vi "Resolve Direction Position.vi"(7 "Board Size":i32, 10 "Direction":T1, 11 "From":T2) -> (2 "Col":i32, 3 "Row":i32, 5 "To":T2)   [LabVIEW 2020, in "SquareBattle.lvlib"]
uses:
  SquareBattle.lvlib
  Position.ctl
  Direction.ctl
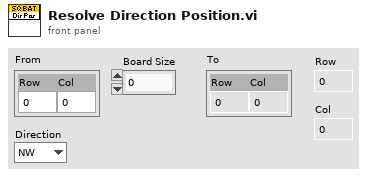
[diagram p1: front panel]
types:
  T1 = typedef "SquareBattle.lvlib/Direction.ctl" = enum16{"NW", "N", "NE", "E", "SE", "S", "SW", "W"}
  T2 = typedef "SquareBattle.lvlib/Position.ctl" = cluster{"Row":i32, "Col":i32}
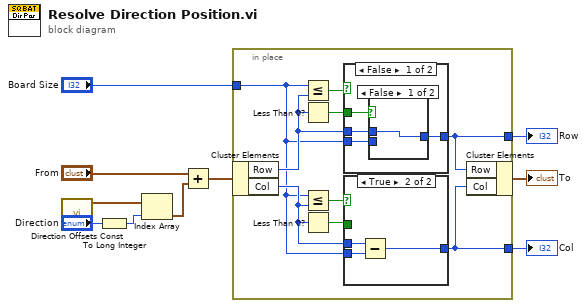
[diagram p0: block diagram]
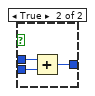
[diagram p3: hidden frame]
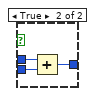
[diagram p4: hidden frame]
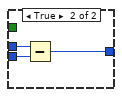
[diagram p5: hidden frame]
diagram:
  n1 = call "Direction Offsets Const.vi"() -> ("Direction Offsets"=w9:T2[])  [unwired: 11 in]
  n2 = To Long Integer(number="Direction") -> (32bit integer=w8:i32)
  n3 = Index Array(array=w9, index=w8) -> (element=w7:T2)
  n4 = Add(x="From", y=w7) -> (x+y=w5:T2)
  n5 = in-place {
    in-place-border: "Board Size" -> [w13]
    in-place-border: [w12] -> w2
    in-place-border: [w11] -> w1
    n6 = in-place-cluster #1(w5) -> ("Row"=w17:i32, "Col"=w14:i32)
    n7 = Less Or Equal?(x=w13, y=w17) -> (x <= y?=w19:bool)
    n8 = Less Than 0?(x=w17) -> (x < 0?=w18:bool)
    n9 = Less Or Equal?(x=w13, y=w14) -> (x <= y?=w16:bool)
    n10 = Less Than 0?(x=w14) -> (x < 0?=w15:bool)
    n11 = case shown="False" w19 {
      tunnel: w18 -> [w34 _]
      tunnel: w17 -> [w33 w41]
      tunnel: w13 -> [w32 w40]
      tunnel: [w31 w39] -> w11
      frame False {
        n12 = case shown="False" w34 {
          tunnel: w33 -> [w35 w38]
          tunnel: w32 -> [_ w37]
          tunnel: [w35 w36] -> w31
          frame False {
          }
          frame True {
            n13 = Add(x=w38, y=w37) -> (x+y=w36:i32)
          }
        }
      }
      frame True {
        n14 = Subtract(x=w41, y=w40) -> (x-y=w39:i32)
      }
    }
    n15 = case shown="True" w16 {
      tunnel: w15 -> [w23 _]
      tunnel: w14 -> [w22 w30]
      tunnel: w13 -> [w21 w29]
      tunnel: [w20 w28] -> w12
      frame False {
        n16 = case shown="False" w23 {
          tunnel: w22 -> [w24 w27]
          tunnel: w21 -> [_ w26]
          tunnel: [w24 w25] -> w20
          frame False {
          }
          frame True {
            n17 = Add(x=w27, y=w26) -> (x+y=w25:i32)
          }
        }
      }
      frame True {
        n18 = Subtract(x=w30, y=w29) -> (x-y=w28:i32)
      }
    }
    n19 = in-place-cluster #1("Row"=w11, "Col"=w12) -> (→"To":T2)
  }
  "Col" <- w2
  "Row" <- w1
